vi "FTW-Package-Lossy-Construct.vi"(9 "max queue size (1)":i32=1, 11 "error in":errorcluster) -> (4 "FTW-Message-Lossy":refnum<class "FTW-Package-Lossy.lvclass">, 15 "error out":errorcluster)   [LabVIEW 2013, in "FTW-Package-Lossy.lvclass"]
uses:
  FTW-Package-Lossy.lvclass
  FTW-Package-Lossy.lvclass/FTW-Package-Lossy.ctl
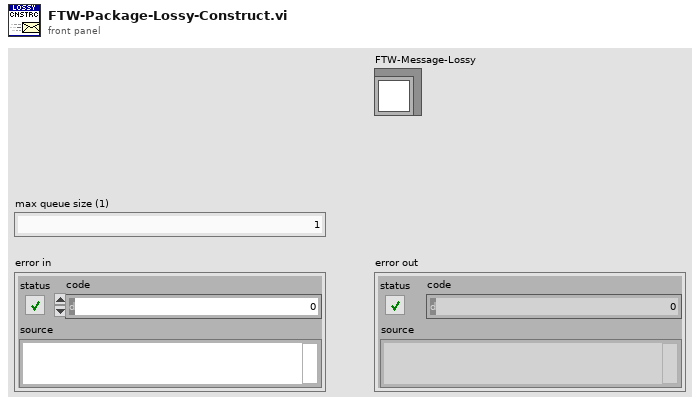
[diagram p1: front panel]
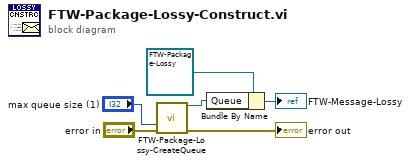
[diagram p0: block diagram]
diagram:
  n1 = call "FTW-Package-Lossy-CreateQueue.vi"("max queue size (1)"="max queue size (1)", "error in"="error in") -> ("Queue"=w4:refnum<queue>, "error out"=→"error out":errorcluster)  [unwired: 12 in]
  n2 = Bundle By Name(cluster=refnum<class "FTW-Package-Lossy.lvclass"> refnum ("FTW-Message-Lossy"), "Queue"=w4) -> (→"FTW-Message-Lossy":refnum<class "FTW-Package-Lossy.lvclass">)
